vi "Main.vi"() -> ()   [LabVIEW 2023]
doc: "This template is for the Queued Message Handler design pattern.\n\nThe Event Handling Loop generates messages based on user interface actions.\n\nThe Message Handling Loop processes messages generated by the Event Handling Loop, or by other messages. The messages are string values, so new messages can be added easily to the Message Cases case structure in the Message Handling Loop. Each message cluster can also provide an optional value for Message Data, which is a variant that can be converted to whatever message-specific data is required."
uses:
  PIDModBus/Controls/PID Cluster.ctl
  controls/VNALogOpt.ctl
  LibreVNA/Types/Trace Enum.ctl
  <vilib>/Utility/error.llb/Trim Whitespace One-Sided.vi
  support/Message Queue/Enqueue Message (Single).vi
  <vilib>/NI/Modbus Library/API/Master/Modbus Master.lvclass
  LibreVNA/LibreVNA.lvclass
  support/Message Queue/Message Queue.lvlib
  support/User Event - Stop/User Event - Stop.lvlib
  PIDModBus/PIDModbus.lvlib
panel:
  out "AppExit":bool
  in  "Tab Control":T1(tab)
  out "Temperature":cluster{"Temperature (C)":dbl, "Value":dbl}(graph)
  out "Output":bool
  out "Output (%)":dbl format="%4.1f %%"
  out "S-Parameter":cluster{"S-Param":dbl[], dbl[]}(graph)
  out "VNA":bool
  in  "btnConnectVNA":bool
  in  "btnMeasureSParam":bool
  in  "VNALogOpt":T2={"VNALogSelect"=enum."No Selection", "VNALogTIncr"=5.0, "VNALogTList"=""} caption="VNA Log Option" {"VNALogTIncr" min=1.0 step=1.0 format="%#.1g"}
  in  "File Path":path=path "C:/Temp"
  in  "LogData":bool
  in  "PartName":string="Unnamed"
  out "Mesg":string
  out "Thermometer":dbl(slide) scale=0.0..150.0
  out "Register Reading":u16
  in  "PID":T3
  out "Boolean":bool
  in  "btnReadReg 2":bool
  in  "Value":u16 format="%x"
  in  "btnReadReg":bool
  in  "Register":u16 format="%x"
  in  "btnSetPID":bool
  in  "btnSetSP":bool
  in  "Set Point (C)":dbl
  in  "btnConnect":bool
  in  "VISA resource":refnum<visa-resource-name>
  in  "Exit":bool
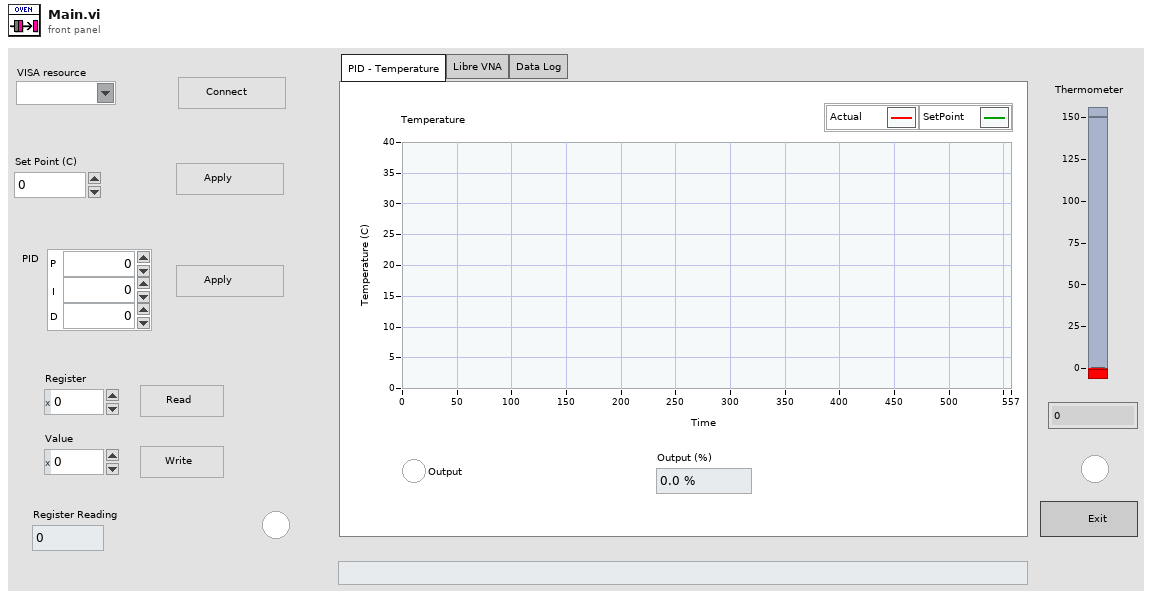
[diagram p1: front panel]
types:
  T1 = enum32{"PID - Temperature", "Libre VNA", "Data Log"}
  T2 = typedef "VNALogOpt.ctl" = cluster{"VNALogSelect":enum32{"No Selection", "TempIncr", "TempList"}, "VNALogTIncr":dbl, "VNALogTList":string}
  T3 = typedef "PIDModbus.lvlib/PID Cluster.ctl" = cluster{"P":u16, "I":u16, "D":u16}
  T4 = enum8{"Enabled", "Disabled", "Disabled and Grayed Out"}
  T5 = typedef "LibreVNA.lvclass/Trace Enum.ctl" = enum16{"S11", "S12", "S21", "S22"}
  T6 = enum32{"invalid app kind", "Development System", "Run Time System", "Student Edition", "Embedded LabVIEW", "Evaluation", "Custom"}
  T7 = typedef "Message Queue.lvlib/All Message Queues.ctl" = cluster{"UI":refnum<queue>}
  T8 = typedef "UI Data.ctl" = cluster{"session":refnum<class "Modbus Master.lvclass">, "IsOpen":bool, "Timeout (ms)":i32, "TempFile":path, "LogStartTime":timestamp, "LibreVNA":refnum<class "LibreVNA.lvclass">, "VNAOpen":bool, "TempSP":dbl, "ActualTemp":dbl, "FileSaved":bool, "PIDOutput":dbl, "VNALogOpt":refnum<vi>, "PartName":string, "ComPort":refnum<visa-resource-name>, "S-Param Data":dbl[][], "VNADataFile - TDMS":path}
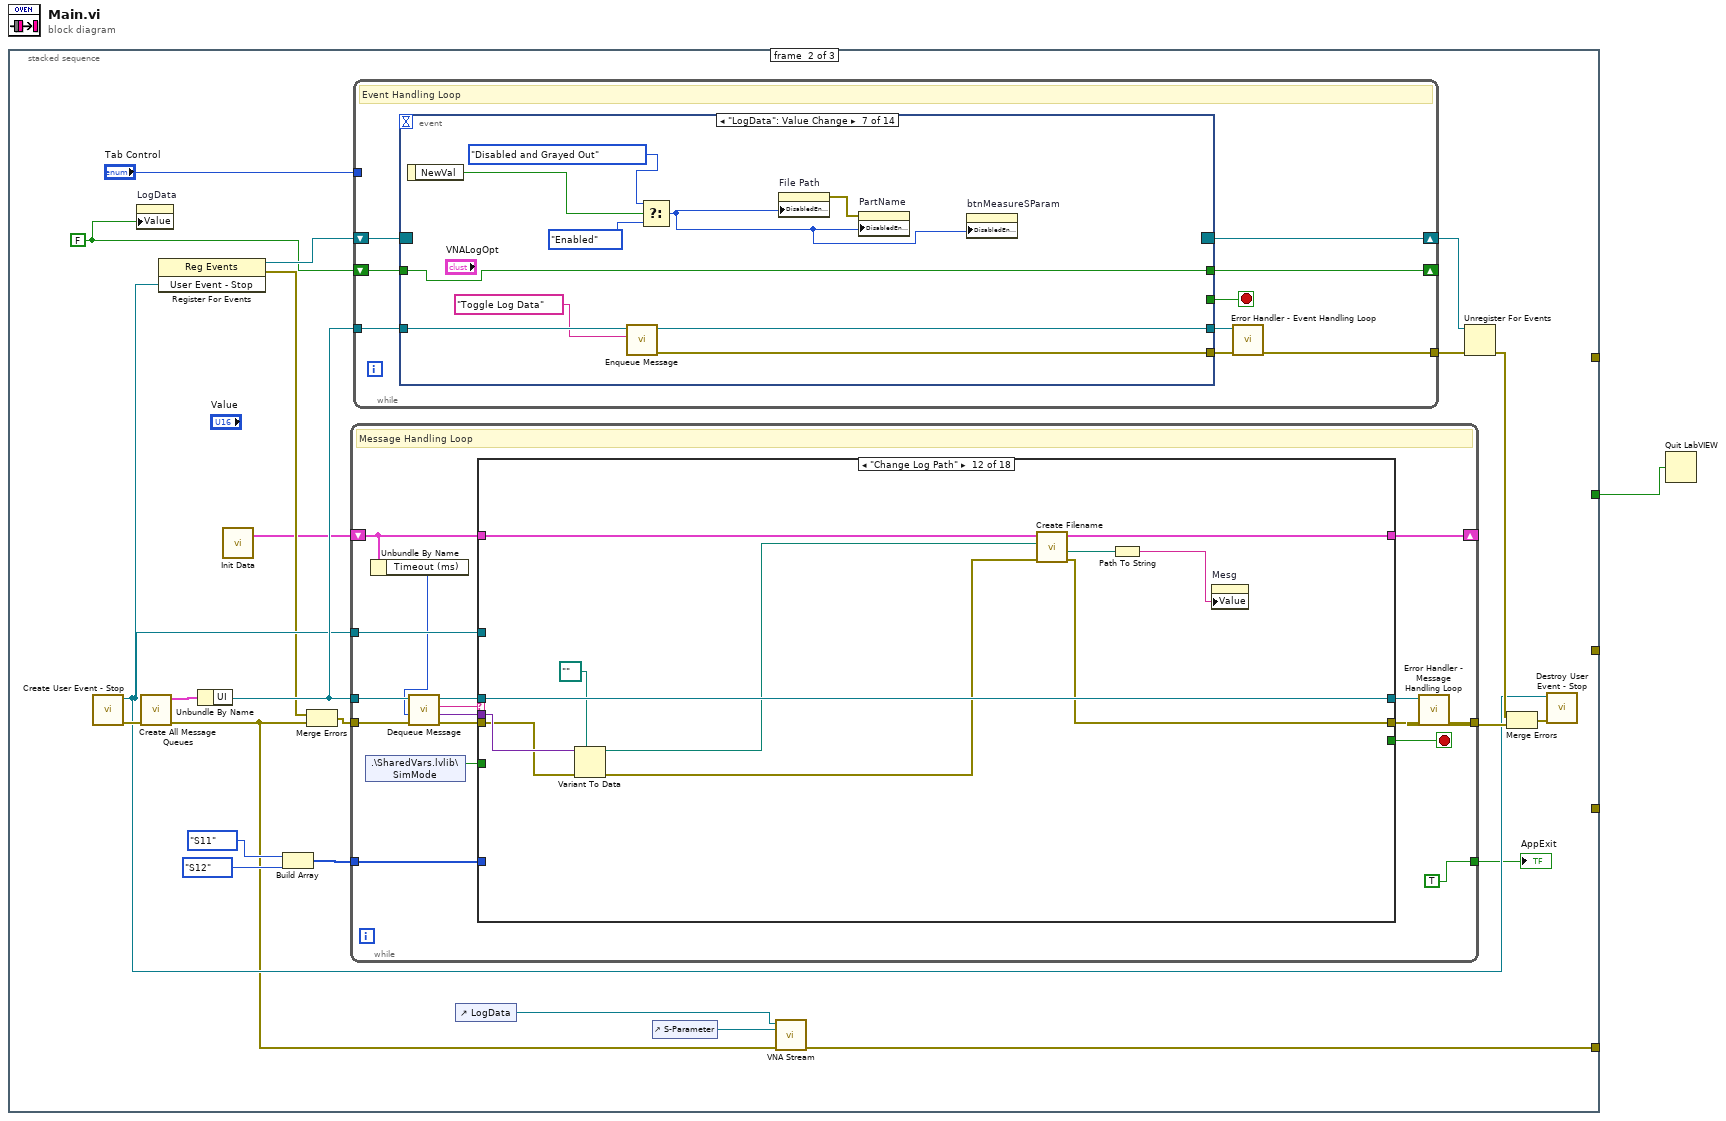
[diagram p0: block diagram]
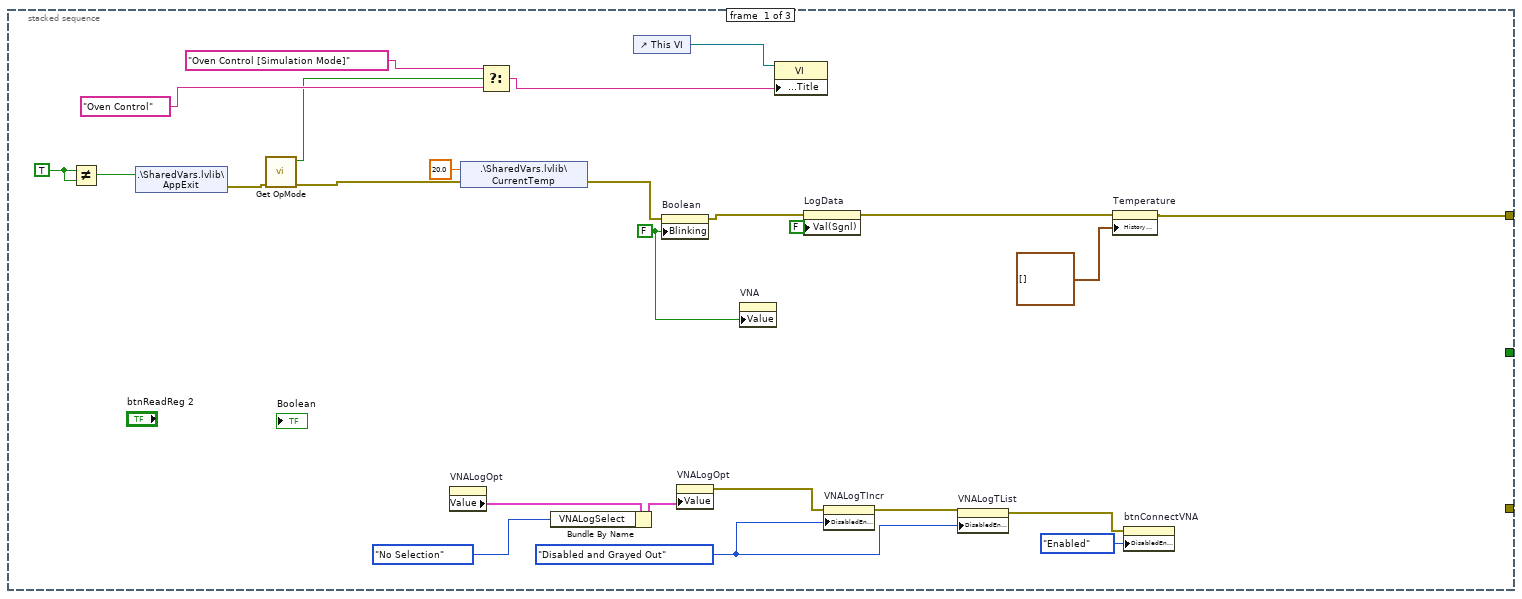
[diagram p2: hidden frame]
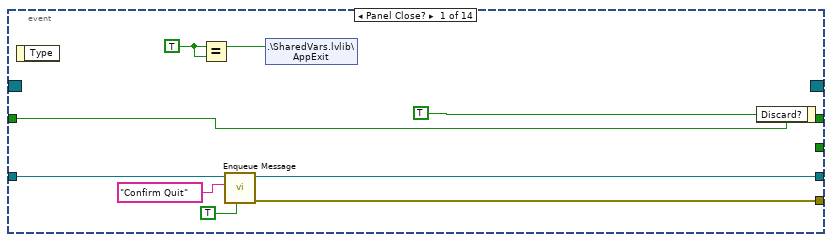
[diagram p3: hidden frame]
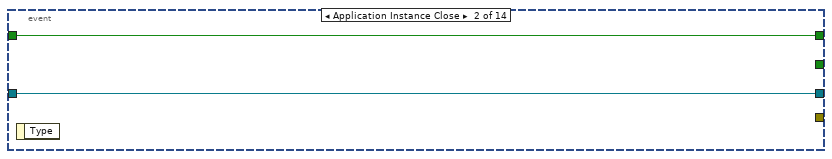
[diagram p4: hidden frame]
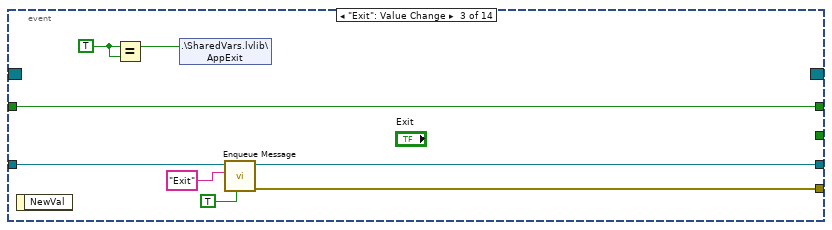
[diagram p5: hidden frame]
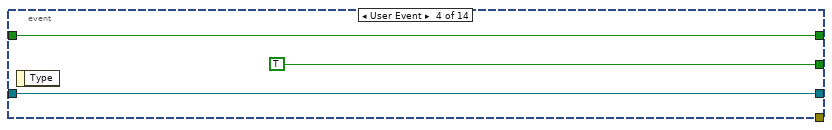
[diagram p6: hidden frame]
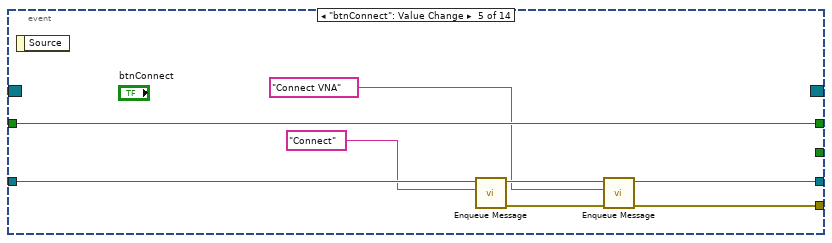
[diagram p7: hidden frame]
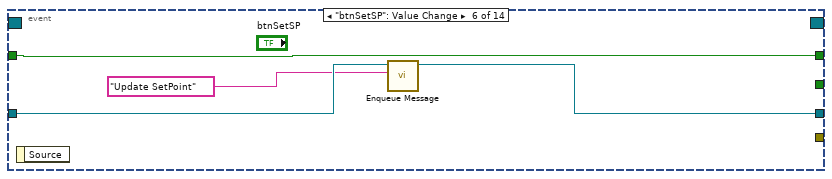
[diagram p8: hidden frame]
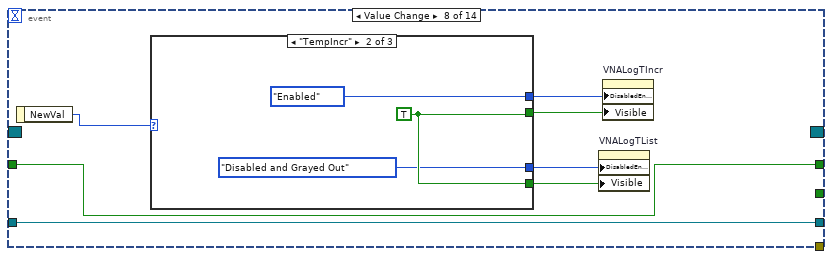
[diagram p9: hidden frame]
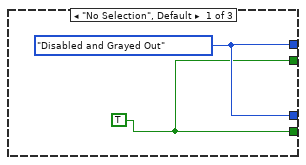
[diagram p10: hidden frame]
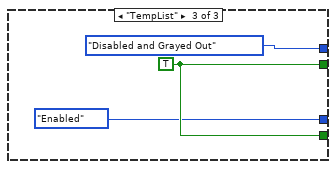
[diagram p11: hidden frame]
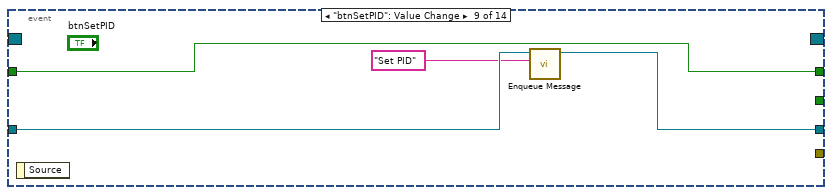
[diagram p12: hidden frame]
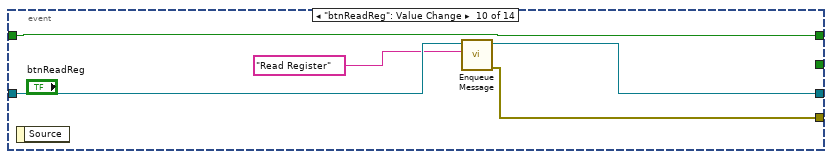
[diagram p13: hidden frame]
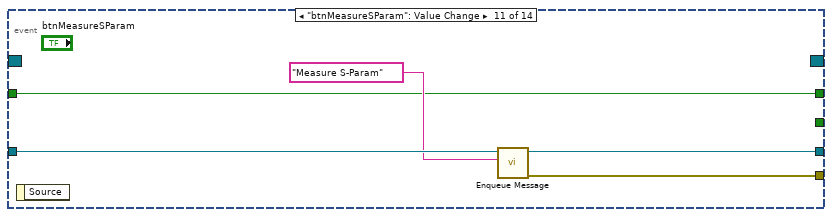
[diagram p14: hidden frame]
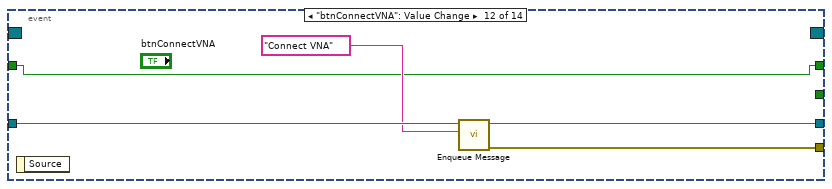
[diagram p15: hidden frame]
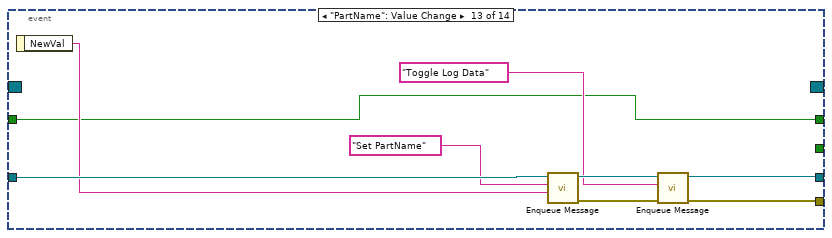
[diagram p16: hidden frame]
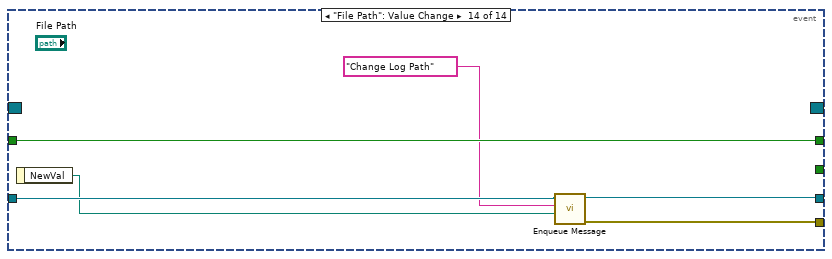
[diagram p17: hidden frame]
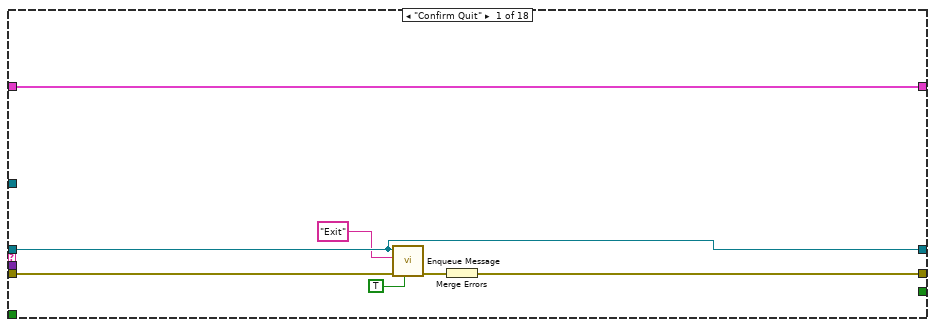
[diagram p18: hidden frame]
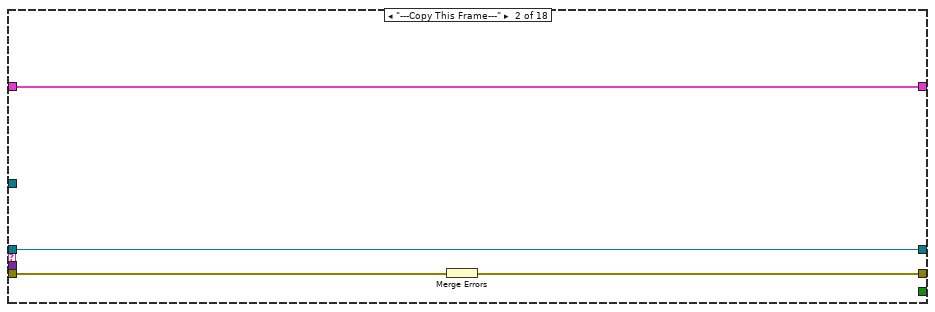
[diagram p19: hidden frame]
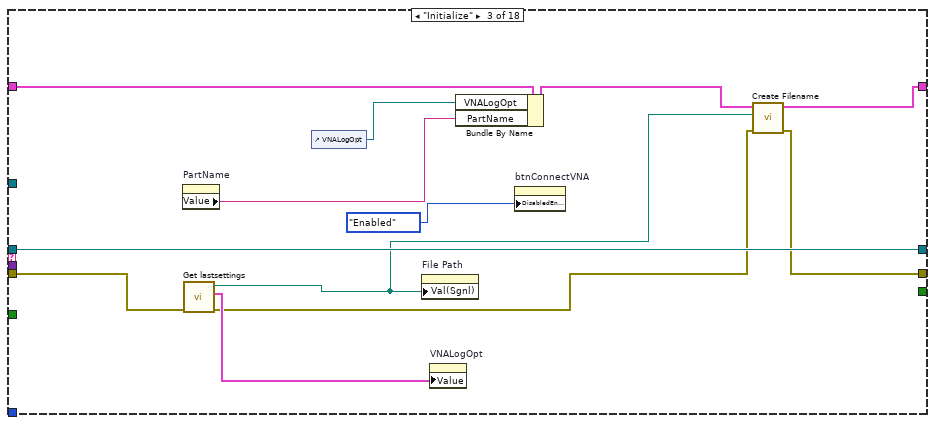
[diagram p20: hidden frame]
diagram:
  n1 = stacked-sequence {
    tunnel: [w25 _ _] -> _
    tunnel: [_ _ w425] -> w1
    tunnel: [_ _ w424] -> _
    tunnel: [_ _ w419] -> _
    tunnel: [_ w28 _] -> _
    frame #0 {
      w5 = TRUE ("AppExit")
      w16 = T4."Disabled and Grayed Out" ("Disabled")
      w21 = FALSE ("Blinking")
      n2 = Not Equal?(x=w5, y=w5) -> (x != y?=w6:bool)
      n3 = shared-variable ".\\SharedVars.lvlib\\AppExit"(w6) -> (error out=w4:errorcluster)  [unwired: 1 in]
      n4 = call "Get OpMode.vi"("error in (no error)"=w4) -> ("error out"=w12:errorcluster, "SimMode"=w7:bool)  [unwired: 5 in]
      n5 = property on="VNALogOpt" class="Clust (strict)"() -> ("Value"=w20:T2)  [unwired: 2 in, 2 out]
      n6 = shared-variable ".\\SharedVars.lvlib\\CurrentTemp"(20.0 ("CurrentTemp"), error in=w12) -> (error out=w13:errorcluster)
      n7 = Select(t="Oven Control [Simulation Mode]", s=w7, f="Oven Control") -> (s? t:f=w8:string)
      n8 = Bundle By Name(cluster=w20, "VNALogSelect"=enum32{"No Selection", "TempIncr", "TempList"}."No Selection") -> (w19:T2)
      n9 = control-ref of="This VI"() -> (w9:refnum<vi>)
      n10 = property on="Boolean" class="Bool (strict)"(error in=w13, "Blinking"=w21) -> (error out=w22:errorcluster)  [unwired: 1 in, 1 out]
      n11 = property on="VNALogOpt" class="Clust (strict)"("Value"=w19) -> (error out=w17:errorcluster)  [unwired: 2 in, 1 out]
      n12 = property on="VNA" class="Bool (strict)"("Value"=w21) -> ()  [unwired: 2 in, 2 out]
      n13 = property class="VI"(reference=w9, "Front Panel.Title"=w8) -> ()  [unwired: 1 in, 2 out]
      n14 = property on="LogData" class="Bool (strict)"(error in=w22, "Val(Sgnl)"=FALSE ("LogData")) -> (error out=w23:errorcluster)  [unwired: 1 in, 1 out]
      n15 = property on="VNALogTIncr" class="DigNum (strict)"(error in=w17, "DisabledEnum"=w16) -> (error out=w15:errorcluster)  [unwired: 1 in, 1 out]
      n16 = property on="VNALogTList" class="Str"(error in=w15, "DisabledEnum"=w16) -> (error out=w3:errorcluster)  [unwired: 1 in, 1 out]
      n17 = property on="Temperature" class="WFChart (strict)"(error in=w23, "History Data"=cluster{"Temperature (C)":dbl, "Value":dbl}[] []) -> (error out=w25:errorcluster)  [unwired: 1 in, 1 out]
      n18 = property on="btnConnectVNA" class="Bool"(error in=w3, "DisabledEnum"=T4."Enabled" ("Disabled")) -> ()  [unwired: 1 in, 2 out]
    }
    frame #1 {
      w32 = FALSE ("LogData")
      n19 = call "Create User Event - Stop.vi"() -> ("error out"=w46:errorcluster, "User Event - Stop"=w40:refnum<user-event>)  [unwired: 10 in]
      n20 = property on="LogData" class="Bool (strict)"("Value"=w32) -> ()  [unwired: 2 in, 2 out]
      n21 = call "Create All Message Queues.vi"("error in (no error)"=w46) -> ("error out"=w30:errorcluster, "Message Queues out"=w49:T7)  [unwired: 9 in]
      n22 = register-events(w40) -> (reference out=w41:refnum<event-registration>, error out=w38:errorcluster)  [unwired: 2 in]
      n23 = Unbundle By Name(w49) -> ("UI"=w47:refnum<queue>)
      n24 = call "Init Data.vi"() -> ("Data Out"=w37:T8)  [unwired: 11 in]
      n25 = Build Array(Trace_Enum."S11" ("Trace Name"), Trace_Enum."S12" ("Trace Name")) -> (w33:T5[])
      n26 = Merge Errors(w38, w30) -> (w39:errorcluster)
      n27 = while {
        tunnel: w47 -> [w160]
        shift-right: [w167] -> _
        shift-left: w37 -> [w156]
        tunnel: w40 -> [w165]
        tunnel: w39 -> [w164]
        tunnel: [w158] -> w48
        tunnel: w33 -> [w152]
        tunnel: [TRUE] -> w31
        stop <- w166 stop-if-true
        # "Message Handling Loop"
        n28 = shared-variable ".\\SharedVars.lvlib\\SimMode"() -> (w153:bool)  [unwired: 1 in, 1 out]
        n29 = Unbundle By Name(w156) -> ("Timeout (ms)"=w155:i32)
        n30 = call "Dequeue Message.vi"("error in (no error)"=w164, "timeout in ms (-1)"=w155, "Message Queue"=w160) -> ("error out"=w163:errorcluster, "Message Data"=w161:variant, "Message"=w162:string, "dup Message Queue"=w159:refnum<queue>)  [unwired: 5 in]
        n31 = case "Message Cases" shown="\"Change Log Path\"" w162 {
          tunnel: w159 -> [w170 w175 w188 w194 w216 w238 w249 w278 w303 w314 w322 w339 w348 w357 w363 w369 w387 w391]
          tunnel: w163 -> [w174 w178 w186 w202 w212 w236 w255 w283 w294 w309 w323 w332 _ w349 w364 w366 w381 w393]
          tunnel: [w172 w176 w180 w195 w211 w228 w252 w279 w286 w308 w320 w336 w347 w349 w364 w368 w384 w394] -> w157
          tunnel: w156 -> [w173 w177 w190 w204 w215 w239 w257 w285 w302 w313 w324 w338 w345 w351 w362 w370 w377 w397]
          tunnel: [w173 w177 w182 w201 w214 w231 w251 w282 w290 w307 w315 w337 w345 w351 w360 w370 w377 w395] -> w167
          tunnel: [_ _ _ _ _ _ _ _ _ _ _ _ _ _ _ _ TRUE _] -> w166
          tunnel: w161 -> [_ _ _ _ _ w237 _ _ _ _ _ w335 _ _ _ w367 w378 _]
          tunnel: w165 -> [_ _ _ _ _ _ _ _ _ _ _ _ _ _ _ _ w383 _]
          tunnel: [w170 w175 w188 w194 w216 w238 w249 w277 w303 w314 w321 w339 w348 w357 w363 w369 w387 w390] -> w154
          tunnel: w153 -> [_ _ _ w191 _ _ _ _ _ _ w316 _ _ _ _ _ _ _]
          tunnel: w152 -> [_ _ _ _ _ _ _ _ _ _ _ _ _ _ _ _ _ w388]
          frame "Confirm Quit" {
            # "Confirm Quit - Message that can confirm whether or not the user wants to exit the application."
            n32 = call-poly "Enqueue Message.vi"("Priority Message? (F)"=TRUE, "error in (no error)"=w174, "Message"="Exit", "Message Queue"=w170) -> ("error out"=w171:errorcluster)  [unwired: 6 in, 1 out]
            n33 = Merge Errors(w171) -> (w172:errorcluster)
          }
          frame "---Copy This Frame---" {
            # "Duplicate this frame when creating new messages.  Change this comment in the duplicated frame to describe this message."
            n34 = Merge Errors(w178) -> (w176:errorcluster)
          }
          frame "Initialize" {
            # "Duplicate this frame when creating new messages.  Change this comment in the duplicated frame to describe this message."
            n35 = property on="PartName" class="Str"() -> ("Value"=w184:string)  [unwired: 2 in, 2 out]
            n36 = call "Get lastsettings.vi"("error in"=w186) -> ("error out"=w181:errorcluster, "VNALogOpt"=w185:T2, "Path"=w179:path)  [unwired: 4 in]
            n37 = control-ref of="VNALogOpt"() -> (w189:refnum<vi>)
            n38 = property on="File Path" class="Path"("Val(Sgnl)"=w179) -> ()  [unwired: 2 in, 2 out]
            n39 = property on="VNALogOpt" class="Clust (strict)"("Value"=w185) -> ()  [unwired: 2 in, 2 out]
            n40 = Bundle By Name(cluster=w190, "VNALogOpt"=w189, "PartName"=w184) -> (w183:T8)
            n41 = property on="btnConnectVNA" class="Bool"("DisabledEnum"=T4."Enabled" ("f")) -> ()  [unwired: 2 in, 2 out]
            n42 = call "Create Filename.vi"("error in"=w181, "Path in"=w179, "Data in"=w183) -> ("error out"=w180:errorcluster, "Data Out"=w182:T8)  [unwired: 6 in, 1 out]
          }
          frame "Connect" {
            # "Duplicate this frame when creating new messages.  Change this comment in the duplicated frame to describe this message."
            n43 = case shown="False" w191 {
              tunnel: "VISA resource" -> [w208 _]
              tunnel: w202 -> [w207 w209]
              tunnel: [w206 _] -> w200
              tunnel: [w205 w209] -> w196
              frame False {
                n44 = call "Initialize.vi"("error in (no error)"=w207, "VISA resource name"=w208) -> ("error out"=w205:errorcluster, "session out"=w206:refnum<class "Modbus Master.lvclass">)  [unwired: 8 in]
              }
              frame True {
              }
            }
            n45 = Not(x=w196) -> (.not. x?=w192:bool)
            n46 = Select(t=50, s=w192, f=-1 ("Timeout (ms)")) -> (s? t:f=w197:i32)
            n47 = call-poly "Enqueue Message.vi"("error in (no error)"=w196, "Message"="Get Status", "Message Queue"=w194) -> ("error out"=w195:errorcluster)  [unwired: 7 in, 1 out]
            n48 = Bundle By Name(cluster=w204, "session"=w200, "IsOpen"=w192, "Timeout (ms)"=w197) -> (w201:T8)
          }
          frame "Update SetPoint" {
            n49 = Unbundle By Name(w215) -> ("IsOpen"=w210:bool)
            n50 = case shown="True" w210 {
              tunnel: w215 -> [w218 w225]
              tunnel: [w218 w223] -> w214
              tunnel: "Set Point (C)" -> [_ w219]
              tunnel: w212 -> [w217 w221]
              tunnel: [w217 w220] -> w211
              frame False {
              }
              frame True {
                n51 = Unbundle By Name(w225) -> ("session"=w224:refnum<class "Modbus Master.lvclass">)
                n52 = call "Set TempSP.vi"("error in (no error)"=w221, "Temp SP(C)"=w219, "Modbus Master in"=w224) -> ("error out"=w220:errorcluster, "Modbus Master out"=w222:refnum<class "Modbus Master.lvclass">)  [unwired: 7 in]
                n53 = Bundle By Name(cluster=w225, "session"=w222, "TempSP"=w219) -> (w223:T8)
              }
            }
          }
          frame "Set PartName" {
            n54 = Variant To Data(error in=w236, type="", Variant=w237) -> (data=w234:string, error out=w229:errorcluster)
            n55 = call <vilib>:"Trim Whitespace.vi"("string"=w234) -> ("trimmed string"=w233:string)  [unwired: 1 in]
            n56 = Bundle By Name(cluster=w239, "PartName"=w233) -> (w232:T8)
            n57 = property on="File Path" class="Path"() -> ("Value"=w230:path)  [unwired: 2 in, 2 out]
            n58 = call "Create Filename.vi"("error in"=w229, "Path in"=w230, "Data in"=w232) -> ("error out"=w228:errorcluster, "TDMS FileName"=w227:path, "Data Out"=w231:T8)  [unwired: 6 in]
            n59 = Path To String(path=w227) -> (string=w226:string)
            n60 = property on="Mesg" class="Str"("Value"=w226) -> ()  [unwired: 2 in, 2 out]
          }
          frame "Get Status" {
            n61 = Unbundle By Name(w257) -> ("session"=w256:refnum<class "Modbus Master.lvclass">)
            n62 = call "Get PID Values.vi"("error in (no error)"=w255, "Modbus Master in"=w256) -> ("error out"=w253:errorcluster, "register values"=w250:dbl[], "Modbus Master out"=w254:refnum<class "Modbus Master.lvclass">)  [unwired: 7 in]
            n63 = To Unsigned Word Integer(number=w250) -> (unsigned 16bit integer=w247:u16[])
            n64 = Index Array(array=w247) -> (element #1=w245:u16, element #2=w244:u16, element #3=w243:u16)  [unwired: 3 in]
            n65 = shared-variable ".\\SharedVars.lvlib\\SimMode"() -> (w241:bool)  [unwired: 1 in, 1 out]
            n66 = call "Get TempSP.vi"("error in (no error)"=w253, "Modbus Master in"=w254) -> ("error out"=w252:errorcluster, "SetPoint (C)"=w242:dbl, "Modbus Master out"=w240:refnum<class "Modbus Master.lvclass">)  [unwired: 7 in]
            n67 = Bundle By Name(cluster=T3 {"P"=0, "I"=0, "D"=0} ("PID"), "P"=w245, "I"=w244, "D"=w243) -> (w246:T3)
            n68 = property on="PID" class="Clust (strict)"("Value"=w246) -> ()  [unwired: 2 in, 2 out]
            n69 = case shown="False" w241 {
              tunnel: w257 -> [w261 w265]
              tunnel: [w260 w264] -> w251
              tunnel: w240 -> [w259 _]
              tunnel: w242 -> [w258 _]
              tunnel: w240 -> [_ w263]
              frame False {
                n70 = Bundle By Name(cluster=w261, "session"=w259, "TempSP"=w258) -> (w260:T8)
                n71 = property on="Set Point (C)" class="DigNum (strict)"("Value"=w258) -> ()  [unwired: 2 in, 2 out]
              }
              frame True {
                n72 = property on="Set Point (C)" class="DigNum (strict)"() -> ("Value"=w262:dbl)  [unwired: 2 in, 2 out]
                n73 = Bundle By Name(cluster=w265, "session"=w263, "TempSP"=w262) -> (w264:T8)
              }
            }
          }
          frame "Connect VNA" {
            n74 = Unbundle By Name(w285) -> ("LibreVNA"=w284:refnum<class "LibreVNA.lvclass">)
            n75 = call-dynamic "Open.vi"("error in (no error)"=w283, "LibreVNA in"=w284) -> ("error out"=w280:errorcluster, "LibreVNA out"=w281:refnum<class "LibreVNA.lvclass">)  [unwired: 8 in]
            n76 = call-dynamic "Read IsOpen.vi"("error in (no error)"=w280, "LibreVNA in"=w281) -> ("error out"=w271:errorcluster, "IsOpen"=w268:bool, "LibreVNA out"=w273:refnum<class "LibreVNA.lvclass">)  [unwired: 7 in]
            "VNA" <- w268
            n77 = call "VNA ContinuousRun.vi"("error in (no error)"=w271, "LibreVNA in"=w273) -> ("error out"=w270:errorcluster, "LibreVNA out"=w272:refnum<class "LibreVNA.lvclass">)  [unwired: 8 in]
            n78 = call-dynamic "VNA Start Run.vi"("error in (no error)"=w270, "LibreVNA in"=w272) -> ("error out"=w275:errorcluster, "LibreVNA out"=w274:refnum<class "LibreVNA.lvclass">)  [unwired: 7 in, 1 out]
            n79 = Bundle By Name(cluster=w285, "LibreVNA"=w274, "VNAOpen"=w268) -> (w282:T8)
            n80 = Select(t=T4."Disabled and Grayed Out", s=w268, f=T4."Enabled" ("Disabled")) -> (s? t:f=w266:T4)
            n81 = call-poly "Enqueue Message.vi"("error in (no error)"=w275, "Message"="Set VNA Log Option", "Message Queue"=w278) -> ("error out"=w279:errorcluster, "dup Message Queue"=w277:refnum<queue>)  [unwired: 7 in]
            n82 = property on="btnConnectVNA" class="Bool"("DisabledEnum"=w266) -> ()  [unwired: 2 in, 2 out]
          }
          frame "Measure S-Param" {
            n83 = property on="File Path" class="Path"() -> ("Value"=w301:path)  [unwired: 2 in, 2 out]
            n84 = property on="Mesg" class="Str"(error in=w294, "Value"="") -> (error out=w293:errorcluster)  [unwired: 1 in, 1 out]
            n85 = call "Measure S-Param.vi"("error in (no error)"=w293, "DataFile"=w301, "Data in"=w302) -> ("error out"=w287:errorcluster, "FileSaved"=w300:bool, "Data Out out"=w291:T8)  [unwired: 2 in]
            n86 = Path To String(path=w301) -> (string=w299:string)
            n87 = Concatenate Strings("Data is saved to " ("string"), w299) -> (w296:string)
            n88 = Select(t=w296, s=w300, f="") -> (s? t:f=→"Mesg":string)
            n89 = call "Get S-Param Mag.vi"("error in"=w287, "Trace Name"=Trace_Enum."S12", "Data in"=w291) -> ("error out"=w286:errorcluster, "Graph"=→"S-Parameter":cluster{"Array":dbl[], "Array":dbl[]}, "Data Out"=w290:T8)  [unwired: 1 in, 1 out]
          }
          frame "Read Register" {
            n90 = Unbundle By Name(w313) -> ("session"=w312:refnum<class "Modbus Master.lvclass">)
            n91 = call-dynamic "Read Holding Registers.vi"("error in"=w309, "number of inputs"=u16 1, "starting address"="Register", "Modbus master in"=w312) -> ("error out"=w308:errorcluster, "register values"=w305:u16[], "Modbus master out"=w306:refnum<class "Modbus Master.lvclass">)  [unwired: 5 in]
            n92 = Index Array(array=w305) -> (element=w304:u16)  [unwired: 1 in]
            "Register Reading" <- w304
            n93 = Bundle By Name(cluster=w313, "session"=w306) -> (w307:T8)
            n94 = property on="Value" class="DigNum (strict)"("Value"=w304) -> ()  [unwired: 2 in, 2 out]
          }
          frame "Toggle Log Data" {
            n95 = Bundle By Name(cluster=w324, "PartName"="PartName") -> (w318:T8)
            n96 = case shown="True" w316 {
              tunnel: w318 -> [w325 w328]
              tunnel: [w325 w327] -> w315
              frame False {
              }
              frame True {
                n97 = Bundle By Name(cluster=w328, "Timeout (ms)"=1000) -> (w327:T8)
              }
            }
            n98 = call-poly "Enqueue Message.vi"("error in (no error)"=w323, "Message"="Set VNA Log Option", "Message Queue"=w322) -> ("error out"=w320:errorcluster, "dup Message Queue"=w321:refnum<queue>)  [unwired: 7 in]
          }
          frame "Change Log Path" {
            n99 = Variant To Data(error in=w332, type=path "", Variant=w335) -> (data=w333:path, error out=w331:errorcluster)
            n100 = call "Create Filename.vi"("error in"=w331, "Path in"=w333, "Data in"=w338) -> ("error out"=w336:errorcluster, "TDMS FileName"=w330:path, "Data Out"=w337:T8)  [unwired: 6 in]
            n101 = Path To String(path=w330) -> (string=w329:string)
            n102 = property on="Mesg" class="Str"("Value"=w329) -> ()  [unwired: 2 in, 2 out]
          }
          frame "Set VNA Log Option" {
            n103 = Unbundle By Name(w345) -> ("VNAOpen"=w344:bool)
            n104 = property on="LogData" class="Bool (strict)"() -> ("Value"=w346:bool)  [unwired: 2 in, 2 out]
            n105 = And(x=w344, y=w346) -> (x .and. y?=w343:bool)
            n106 = Select(t=T4."Enabled", s=w343, f=T4."Disabled and Grayed Out") -> (s? t:f=w340:T4)
            n107 = property on="VNALogOpt" class="Clust (strict)"("DisabledEnum"=w340) -> (error out=w347:errorcluster)  [unwired: 2 in, 1 out]
          }
          frame "Check VNA Server" {
            n108 = Unbundle By Name(w351) -> ("VNAOpen"=w350:bool)
            n109 = Select(t=T4."Enabled" ("Disabled"), s=w350, f=T4."Disabled and Grayed Out") -> (s? t:f=w354:T4)
            n110 = property on="VNALogSelect" class="RadioBtnsControl (strict)"("Val(Sgnl)"=enum32{"No Selection", "TempIncr", "TempList"}."No Selection" ("Value (Signaling)")) -> (error out=w352:errorcluster)  [unwired: 2 in, 1 out]
            n111 = property on="VNALogOpt" class="Clust (strict)"(error in=w352, "DisabledEnum"=w354) -> ()  [unwired: 1 in, 2 out]
          }
          frame "Set PID" {
            n112 = Unbundle By Name(w362) -> ("session"=w361:refnum<class "Modbus Master.lvclass">)
            n113 = call "Set PID Values.vi"("PID"="PID", "Modbus Master in"=w361) -> ("Modbus Master out"=w359:refnum<class "Modbus Master.lvclass">)  [unwired: 8 in, 1 out]
            n114 = Bundle By Name(cluster=w362, "session"=w359) -> (w360:T8)
          }
          frame "Error" {
            n115 = Variant To Data(type=w366, Variant=w367) -> (data=w365:errorcluster)  [unwired: 1 in, 1 out]
            n116 = call "Show ErrorMesg.vi"("error in (no error)"=w365) -> ("error out"=w368:errorcluster)  [unwired: 6 in]
          }
          frame "Exit" {
            # "Stop the VI"
            # "Release the message queue reference"
            # "Exit - Exit the application."
            n117 = Variant To Data(type=errorcluster {"status"=FALSE, "code"=0, "source"=""} ("error constant"), Variant=w378) -> (data=w379:errorcluster)  [unwired: 1 in, 1 out]
            n118 = call <vilib>:"Simple Error Handler.vi"("error in (no error)"=w379) -> ()  [unwired: 4 in, 5 out]
            n119 = Unbundle By Name(w377) -> ("LibreVNA"=w373:refnum<class "LibreVNA.lvclass">, "session"=w376:refnum<class "Modbus Master.lvclass">)
            n120 = call "Fire User Event - Stop.vi"("User Event - Stop"=w383) -> ("error out"=w382:errorcluster)  [unwired: 10 in]
            n121 = Release Queue(queue=w387, error in (no error)=w381) -> (error out=w385:errorcluster)  [unwired: 1 in, 2 out]
            n122 = call-dynamic "Shutdown.vi"("Modbus master in"=w376) -> ("error out"=w375:errorcluster)  [unwired: 10 in]
            n123 = Merge Errors(w375, w382, w385) -> (w384:errorcluster)
            n124 = call-dynamic "VNA Stop Run.vi"("LibreVNA in"=w373) -> ("error out"=w371:errorcluster, "LibreVNA out"=w372:refnum<class "LibreVNA.lvclass">)  [unwired: 8 in, 1 out]
            n125 = call-dynamic "Close.vi"("error in (no error)"=w371, "LibreVNA in"=w372) -> ("error out"=w374:errorcluster)  [unwired: 8 in, 1 out]
            n126 = call <vilib>:"Clear Errors.vi"("error in (no error)"=w374) -> ()  [unwired: 5 in, 2 out]
          }
          frame "", Default {
            # "'Default' case only runs if there is a message that isn't defined in any of the other cases.  Output a programming error."
            n127 = Unbundle By Name(w397) -> ("IsOpen"=w392:bool, "session"=w396:refnum<class "Modbus Master.lvclass">, "TempSP"=w389:dbl)
            n128 = case shown="True" w392 {
              tunnel: w397 -> [w400 w418]
              tunnel: w396 -> [_ w417]
              tunnel: [w400 w401] -> w395
              tunnel: [w399 w407] -> w394
              tunnel: w393 -> [w399 w414]
              tunnel: w391 -> [w398 w408]
              tunnel: [w398 w408] -> w390
              tunnel: w389 -> [_ w404]
              tunnel: w388 -> [_ _]
              frame False {
              }
              frame True {
                n129 = call "Get Current Temp.vi"("error in (no error)"=w414, "TempSP"=w404, "Modbus Master in"=w417) -> ("error out"=w411:errorcluster, "Output (V)"=w406:dbl, "Temperature (C)"=w403:dbl, "Modbus Master out"=w415:refnum<class "Modbus Master.lvclass">)  [unwired: 5 in]
                "Thermometer" <- w403
                n130 = property on="LogData" class="Bool (strict)"() -> ("Value"=w410:bool)  [unwired: 2 in, 2 out]
                n131 = property on="Set Point (C)" class="DigNum (strict)"() -> ("Value"=w412:dbl)  [unwired: 2 in, 2 out]
                n132 = Bundle By Name(cluster=w418, "session"=w415, "ActualTemp"=w403, "PIDOutput"=w406) -> (w416:T8)
                n133 = shared-variable ".\\SharedVars.lvlib\\CurrentTemp"(w403) -> ()  [unwired: 1 in, 1 out]
                n134 = Bundle("Temperature (C)"=w403, "Value"=w412) -> (→"Temperature":cluster{"Temperature (C)":dbl, "Value":dbl})  [unwired: 1 in]
                n135 = call "Log Temperature.vi"("error in"=w411, "LogData"=w410, "Data in"=w416) -> ("error out"=w407:errorcluster, "Data Out"=w402:T8)  [unwired: 6 in, 1 out]
                n136 = Unbundle By Name(w402) -> ("PIDOutput"=w405:dbl)
                "Output (%)" <- w405
                n137 = call "AppData - Set.vi"("Data In"=w402) -> ("Data Out"=w401:T8)  [unwired: 5 in, 1 out]
                n138 = Greater Than 0?(x=w405) -> (x > 0?=→"Output":bool)
              }
            }
          }
        }
        n139 = call "Error Handler - Message Handling Loop.vi"("error in (no error)"=w157, "Message Queue"=w154) -> ("dup error in"=w158:errorcluster)  [unwired: 8 in, 1 out]
      }
      "AppExit" <- w31
      n140 = while {
        tunnel: w47 -> [w58]
        shift-right: [w56] -> w43
        shift-left: w41 -> [w57]
        tunnel: [w52] -> w42
        tunnel: "Tab Control" -> [_]
        shift-right: [w51] -> _
        shift-left: w32 -> [w50]
        stop <- w54 stop-if-true
        # "Event Handling Loop"
        n141 = event shown="[6] \"LogData\": Value Change" {
          selector: w57 -> [_ _ _ _ _ _ _ _ _ _ _ _ _ _]
          dyn-events: [_ _ _ _ _ _ _ _ _ _ _ _ _ _] -> w56
          timeout: _ -> [_ _ _ _ _ _ _ _ _ _ _ _ _ _]
          tunnel: [_ _ _ TRUE ("Discard?") _ _ _ _ _ _ _ _ _ _] -> w54
          tunnel: w58 -> [w66 w69 w77 w80 w88 w92 w102 w109 w121 w126 w131 w136 w144 w149]
          tunnel: [w65 _ w76 _ w83 _ w99 _ _ w124 w129 w133 w139 w146] -> w55
          tunnel: [w64 w69 w75 w80 w82 w91 w100 w109 w120 w125 w130 w135 w141 w148] -> w53
          tunnel: [w61 w68 w72 w78 w86 w89 w94 w103 w118 w122 w127 w132 w137 w150] -> w51
          tunnel: w50 -> [w61 w68 w72 w78 w86 w89 w94 w103 w118 w122 w127 w132 w137 w150]
          event Panel Close? {
            w59 = TRUE ("AppExit")
            n142 = event-data() -> ()  [unwired: 1 in, 1 out]
            n143 = Equal?(x=w59, y=w59) -> (x = y?=w60:bool)
            n144 = call-poly "Enqueue Message.vi"("Priority Message? (F)"=TRUE, "Message"="Confirm Quit", "Message Queue"=w66) -> ("error out"=w65:errorcluster, "dup Message Queue"=w64:refnum<queue>)  [unwired: 7 in]
            n145 = shared-variable ".\\SharedVars.lvlib\\AppExit"(w60) -> ()  [unwired: 1 in, 1 out]
            n146 = event-data("Discard?"=TRUE) -> ()  [unwired: 1 in, 1 out]
          }
          event Application Instance Close {
            n147 = event-data() -> ()  [unwired: 1 in, 1 out]
          }
          event "Exit": Value Change {
            w70 = TRUE ("AppExit")
            n148 = event-data() -> ()  [unwired: 1 in, 1 out]
            n149 = Equal?(x=w70, y=w70) -> (x = y?=w71:bool)
            n150 = shared-variable ".\\SharedVars.lvlib\\AppExit"(w71) -> ()  [unwired: 1 in, 1 out]
            n151 = call-poly "Enqueue Message.vi"("Priority Message? (F)"=TRUE, "Message"="Exit", "Message Queue"=w77) -> ("error out"=w76:errorcluster, "dup Message Queue"=w75:refnum<queue>)  [unwired: 7 in]
          }
          event User Event {
            n152 = event-data() -> ()  [unwired: 1 in, 1 out]
          }
          event "btnConnect": Value Change {
            n153 = event-data() -> ()  [unwired: 1 in, 1 out]
            n154 = call-poly "Enqueue Message.vi"("Message"="Connect", "Message Queue"=w88) -> ("error out"=w84:errorcluster, "dup Message Queue"=w85:refnum<queue>)  [unwired: 8 in]
            n155 = call-poly "Enqueue Message.vi"("error in (no error)"=w84, "Message"="Connect VNA", "Message Queue"=w85) -> ("error out"=w83:errorcluster, "dup Message Queue"=w82:refnum<queue>)  [unwired: 7 in]
          }
          event "btnSetSP": Value Change {
            n156 = event-data() -> ()  [unwired: 1 in, 1 out]
            n157 = call-poly "Enqueue Message.vi"("Message"="Update SetPoint", "Message Queue"=w92) -> ("dup Message Queue"=w91:refnum<queue>)  [unwired: 8 in, 1 out]
          }
          event "LogData": Value Change {
            n158 = event-data() -> ("NewVal"=w98:bool)  [unwired: 1 in]
            n159 = call-poly "Enqueue Message.vi"("Message"="Toggle Log Data", "Message Queue"=w102) -> ("error out"=w99:errorcluster, "dup Message Queue"=w100:refnum<queue>)  [unwired: 8 in]
            n160 = Select(t=T4."Disabled and Grayed Out" ("Disabled"), s=w98, f=T4."Enabled") -> (s? t:f=w93:T4)
            n161 = property on="File Path" class="Path"("DisabledEnum"=w93) -> (error out=w95:errorcluster)  [unwired: 2 in, 1 out]
            n162 = property on="PartName" class="Str"(error in=w95, "DisabledEnum"=w93) -> ()  [unwired: 1 in, 2 out]
            n163 = property on="btnMeasureSParam" class="Bool"("DisabledEnum"=w93) -> ()  [unwired: 2 in, 2 out]
          }
          event Value Change {
            n164 = event-data() -> ("NewVal"=w108:enum32{"No Selection", "TempIncr", "TempList"})  [unwired: 1 in]
            n165 = case shown="\"TempIncr\"" w108 {
              tunnel: [w111 T4."Enabled" ("Disabled") T4."Disabled and Grayed Out" ("Disabled")] -> w107
              tunnel: [w111 T4."Disabled and Grayed Out" ("Disabled") T4."Enabled" ("Disabled")] -> w106
              tunnel: [w110 w113 w116] -> w105
              tunnel: [w110 w113 w116] -> w104
              frame "No Selection", Default {
                w110 = TRUE
                w111 = T4."Disabled and Grayed Out" ("Disabled")
              }
              frame "TempIncr" {
                w113 = TRUE
              }
              frame "TempList" {
                w116 = TRUE
              }
            }
            n166 = property on="VNALogTList" class="Str"("DisabledEnum"=w106, "Visible"=w105) -> ()  [unwired: 2 in, 2 out]
            n167 = property on="VNALogTIncr" class="DigNum (strict)"("DisabledEnum"=w107, "Visible"=w104) -> ()  [unwired: 2 in, 2 out]
          }
          event "btnSetPID": Value Change {
            n168 = event-data() -> ()  [unwired: 1 in, 1 out]
            n169 = call-poly "Enqueue Message.vi"("Message"="Set PID", "Message Queue"=w121) -> ("dup Message Queue"=w120:refnum<queue>)  [unwired: 8 in, 1 out]
          }
          event "btnReadReg": Value Change {
            n170 = event-data() -> ()  [unwired: 1 in, 1 out]
            n171 = call-poly "Enqueue Message.vi"("Message"="Read Register", "Message Queue"=w126) -> ("error out"=w124:errorcluster, "dup Message Queue"=w125:refnum<queue>)  [unwired: 8 in]
          }
          event "btnMeasureSParam": Value Change {
            n172 = event-data() -> ()  [unwired: 1 in, 1 out]
            n173 = call-poly "Enqueue Message.vi"("Message"="Measure S-Param", "Message Queue"=w131) -> ("error out"=w129:errorcluster, "dup Message Queue"=w130:refnum<queue>)  [unwired: 8 in]
          }
          event "btnConnectVNA": Value Change {
            n174 = event-data() -> ()  [unwired: 1 in, 1 out]
            n175 = call-poly "Enqueue Message.vi"("Message"="Connect VNA", "Message Queue"=w136) -> ("error out"=w133:errorcluster, "dup Message Queue"=w135:refnum<queue>)  [unwired: 8 in]
          }
          event "PartName": Value Change {
            n176 = event-data() -> ("NewVal"=w142:string)  [unwired: 1 in]
            n177 = call-poly "Enqueue Message.vi"("Message Data"=w142, "Message"="Set PartName", "Message Queue"=w144) -> ("error out"=w140:errorcluster, "dup Message Queue"=w141:refnum<queue>)  [unwired: 7 in]
            n178 = call-poly "Enqueue Message.vi"("error in (no error)"=w140, "Message"="Toggle Log Data", "Message Queue"=w141) -> ("error out"=w139:errorcluster)  [unwired: 7 in, 1 out]
          }
          event "File Path": Value Change {
            n179 = event-data() -> ("NewVal"=w145:path)  [unwired: 1 in]
            n180 = call-poly "Enqueue Message.vi"("Message Data"=w145, "Message"="Change Log Path", "Message Queue"=w149) -> ("error out"=w146:errorcluster, "dup Message Queue"=w148:refnum<queue>)  [unwired: 7 in]
          }
        }
        n181 = call "Error Handler - Event Handling Loop.vi"("error in (no error)"=w55, "Message Queue"=w53) -> ("dup error in"=w52:errorcluster)  [unwired: 8 in, 1 out]
      }
      n182 = control-ref of="LogData"() -> (w27:refnum<vi>)
      n183 = control-ref of="S-Parameter"() -> (w29:refnum<vi>)
      n184 = call "VNA Stream.vi"("error in"=w30, "S-Parameter Graph"=w29, "StreamMode"=w27) -> ("error out"=w28:errorcluster)  [unwired: 8 in]
      n185 = Unregister For Events(event registration refnum=w43, error in=w42) -> (error out=w44:errorcluster)
      n186 = Merge Errors(w44, w48) -> (w45:errorcluster)
      n187 = call "Destroy User Event - Stop.vi"("error in (no error)"=w45, "User Event - Stop"=w40) -> ()  [unwired: 9 in, 1 out]
    }
    frame #2 {
      n188 = property on="Boolean" class="Bool (strict)"("Blinking"=FALSE) -> (error out=w427:errorcluster)  [unwired: 2 in, 1 out]
      n189 = property on="VNA" class="Bool (strict)"(error in=w427, "Value"=FALSE ("VNA")) -> (error out=w426:errorcluster)  [unwired: 1 in, 1 out]
      n190 = property class="App"(error in=w426) -> ("App.Kind"=w429:T6)  [unwired: 1 in, 2 out]
      n191 = Not Equal?(x=w429, y=T6."Development System") -> (x != y?=w425:bool)
      n192 = property on="VNALogOpt" class="Clust (strict)"() -> (error out=w421:errorcluster, "Value"=w422:T2)  [unwired: 2 in, 1 out]
      n193 = property on="File Path" class="Path"(error in=w421) -> (error out=w420:errorcluster, "Value"=w423:path)  [unwired: 1 in, 1 out]
      n194 = call "save current settings.vi"("error in"=w420, "VNALogOpt"=w422, "Path"=w423) -> ("error out"=w424:errorcluster)  [unwired: 4 in]
      n195 = call "MatFIle - Close.vi"() -> ("error out"=w419:errorcluster)  [unwired: 6 in, 1 out]
    }
  }
  n196 = Quit LabVIEW(quit? (T)=w1) -> ()
